vi "XOR Encryption - Stream Cipher.vi"() -> ()   [LabVIEW 2016]
uses:
  <extravilib>/ChannelInstances/Stream-str/Read With Abort.vi
  <extravilib>/ChannelInstances/Stream-str/Write With Abort.vi
  <extravilib>/ChannelInstances/Stream-str/EndpointRead.vi
  <extravilib>/ChannelInstances/Stream-str/Endpoint.vi
  <extravilib>/ChannelInstances/Stream-str/Instantiate.vi
  <extravilib>/ChannelInstances/Stream-str/)Channel.vi
  <resource>/ChannelSupport/_ChannelSupport/WaitIfNeeded.vi
  <extravilib>/ChannelInstances/Stream-str.lvlib
  <vilib>/Analysis/NI_AALBase.lvlib
panel:
  out "min value":u8
  out "max value":u8
  out "Key Distribution":dynamicdata(graph)=[{"t0"=timestamp(0.5 s since 1904-01-01), "dt"=1.0, "Y"=[5.0, 0.0, 5.0, 0.0, 2.0, 0.0, 2.0, 0.0, 3.0, 0.0, 4.0, 0.0, 3.0, 0.0, 1.0, 0.0, 2.0, 0.0, 4.0, 0.0, 6.0, 0.0, 2.0, 0.0, 1.0, 0.0, 1.0, 0.0, 4.0, 0.0, 5.0, 0.0, 5.0, 0.0, 5.0, 0.0, 4.0, 0.0, 1.0, 0.0, 6.0, 0.0, 4.0, 0.0, 5.0, 0.0, 3.0, 0.0, 6.0, 0.0, 2.0, 0.0, 2.0, 0.0, 0.0, 0.0, 3.0, 0.0, 4.0, 0.0, 2.0, 0.0, 4.0, 0.0, 4.0, 0.0, 5.0, 0.0, 2.0, 0.0, 3.0, 0.0, 3.0, 0.0, 0.0, 0.0, 3.0, 0.0, 5.0, 0.0, 1.0, 0.0, 0.0, 0.0, 1.0, 0.0, 6.0, 0.0, 4.0, 0.0, 9.0, 0.0, 7.0, 0.0, 6.0, 0.0, 6.0, 0.0, 5.0, 0.0, 6.0, 0.0, 1.0, 0.0, 8.0, 0.0, 4.0, 0.0, 5.0, 0.0, 3.0, 0.0, 6.0, 0.0, 7.0, 0.0, 7.0, 0.0, 4.0, 0.0, 4.0, 0.0, 0.0, 0.0, 5.0, 0.0, 3.0, 0.0, 1.0, 0.0, 5.0, 0.0, 4.0, 0.0, 2.0, 0.0, 3.0, 0.0, 5.0, 0.0, 5.0, 0.0, 3.0, 0.0, 5.0, 0.0, 1.0, 0.0, 3.0, 0.0, 2.0, 0.0, 3.0, 0.0, 6.0, 0.0, 2.0, 0.0, 4.0, 0.0, 4.0, 0.0, 3.0, 0.0, 1.0, 0.0, 4.0, 0.0, 3.0, 0.0, 3.0, 0.0, 5.0, 0.0, 2.0, 0.0, 1.0, 0.0, 3.0, 0.0, 4.0, 0.0, 3.0, 0.0, 2.0, 0.0, 1.0, 0.0, 4.0, 0.0, 3.0, 0.0, 6.0, 0.0, 2.0, 0.0, 8.0, 0.0, 1.0, 0.0, 4.0, 0.0, 2.0, 0.0, 2.0, 0.0, 2.0, 0.0, 6.0, 0.0, 3.0, 0.0, 2.0, 0.0, 3.0, 0.0, 5.0, 0.0, 2.0, 0.0, 3.0, 0.0, 5.0, 0.0, 3.0, 0.0, 5.0, 0.0, 2.0, 0.0, 1.0, 0.0, 3.0, 0.0, 3.0, 0.0, 3.0, 0.0, 0.0, 0.0, 4.0, 0.0, 4.0, 0.0, 4.0, 0.0, 6.0, 0.0, 3.0, 0.0, 4.0, 0.0, 4.0, 0.0, 1.0, 0.0], "attributes"=variant("NI_ChannelName"=variant(string " (Histogram)"), "NI_ExpIsRelativeTime"=variant(bool TRUE), "NI_ExpStartTimeStamp"=variant(timestamp timestamp(3588586549.4751897 s since 1904-01-01)), "NI_ExpTimeStamp"=variant(timestamp timestamp(3588586549.4751897 s since 1904-01-01)), "NI_ExpXDimension"=variant(string "BIN"), "NI_OriginalChannelName"=variant(string ""))}] caption="Histogram"
  out "Cypher Text":string
  out "Data Out":string
  in  "Plaintext":string
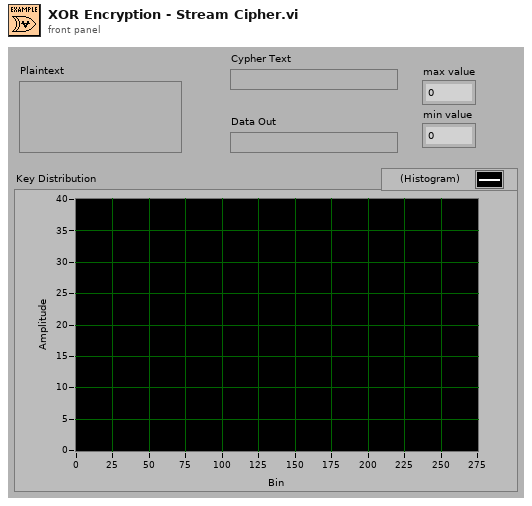
[diagram p1: front panel]
types:
  T1 = typedef "Stream-str.lvlib/)Channel.ctl" = refnum<queue>
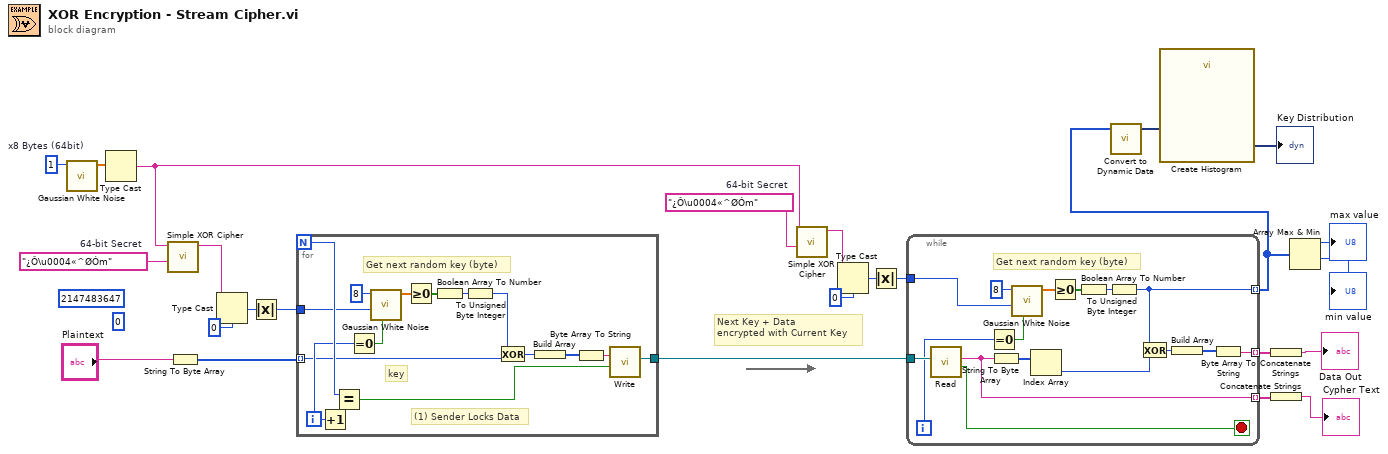
[diagram p0: block diagram]
diagram:
  (unwired) 0 ("seed")
  (unwired) 2147483647 ("seed")
  w14 = "¿Ô\u0004«^ØÓm"  # 64-bit Secret
  w15 = "¿Ô\u0004«^ØÓm"  # 64-bit Secret
  w18 = 1  # x8 Bytes (64bit)
  # "Next Key + Data\nencrypted with Current Key"
  n1 = call <vilib>:"Gaussian White Noise.vi"("samples"=w18) -> ("Gaussian noise pattern"=w17:dbl[])  [unwired: 9 in, 1 out]
  n2 = Type Cast(x=w17) -> (*(type *) &x=w16:string)  [unwired: 1 in]
  n3 = call "Simple XOR Cipher.vi"("key (\"\": random)"=w15, "data in"=w16) -> ("data out"=w13:string)  [unwired: 8 in, 1 out]
  n4 = String To Byte Array(string="Plaintext") -> (unsigned byte array=w22:u8[])
  n5 = Type Cast(type=0 ("seed"), x=w13) -> (*(type *) &x=w11:i32)
  n6 = Absolute Value(x=w11) -> (abs(x)=w7:i32)
  n7 = for {
    N -> [w40]
    tunnel: w22 -> [w34] mode=indexing
    tunnel: [w41] -> w24
    tunnel: w7 -> [w30]
    i -> [w36]
    # "Get next random key (byte)"
    # "key"
    # "(1) Sender Locks Data"
    n8 = Increment(x=w36) -> (x+1=w39:i32)
    n9 = Equal?(x=w40, y=w39) -> (x = y?=w38:bool)
    n10 = Equal To 0?(x=w36) -> (x = 0?=w35:bool)
    n11 = call <vilib>:"Gaussian White Noise.vi"("initialize?"=w35, "seed"=w30, "samples"=8) -> ("Gaussian noise pattern"=w27:dbl[])  [unwired: 7 in, 1 out]
    n12 = Greater Or Equal To 0?(x=w27) -> (x >= 0?=w29:bool[])
    n13 = Boolean Array To Number(Boolean array=w29) -> (number=w28:u32)
    n14 = To Unsigned Byte Integer(number=w28) -> (unsigned 8bit integer=w26:u8)
    n15 = Exclusive Or(1:w34, 2:w26) -> (0:w33:u8)
    n16 = Build Array(w33) -> (w31:u8[])
    n17 = Byte Array To String(unsigned byte array=w31) -> (string=w32:string)
    n18 = call <extravilib>:"Write.vi"("last element? (F)"=w38, "element"=w32) -> ("channel"=w41:T1)  [unwired: 7 in, 2 out]
  }
  n19 = call "Simple XOR Cipher.vi"("key (\"\": random)"=w14, "data in"=w16) -> ("data out"=w9:string)  [unwired: 8 in, 1 out]
  n20 = Type Cast(type=0 ("seed"), x=w9) -> (*(type *) &x=w8:i32)
  n21 = Absolute Value(x=w8) -> (abs(x)=w6:i32)
  n22 = while {
    tunnel: [w49] -> w25 mode=indexing
    tunnel: w24 -> [w57]
    tunnel: [w47] -> w20 mode=indexing
    tunnel: w6 -> [w46]
    tunnel: [w42] -> w3 mode=indexing
    i -> [w48]
    stop <- w56 stop-if-true
    # "Get next random key (byte)"
    n23 = call <extravilib>:"Read.vi"("channel"=w57) -> ("last element?"=w56:bool, "element"=w47:string)  [unwired: 6 in, 3 out]
    n24 = Equal To 0?(x=w48) -> (x = 0?=w54:bool)
    n25 = String To Byte Array(string=w47) -> (unsigned byte array=w51:u8[])
    n26 = call <vilib>:"Gaussian White Noise.vi"("initialize?"=w54, "seed"=w46, "samples"=8) -> ("Gaussian noise pattern"=w45:dbl[])  [unwired: 7 in, 1 out]
    n27 = Index Array(array=w51) -> (element=w50:u8)  [unwired: 1 in]
    n28 = Greater Or Equal To 0?(x=w45) -> (x >= 0?=w44:bool[])
    n29 = Boolean Array To Number(Boolean array=w44) -> (number=w43:u32)
    n30 = To Unsigned Byte Integer(number=w43) -> (unsigned 8bit integer=w42:u8)
    n31 = Exclusive Or(1:w50, 2:w42) -> (0:w53:u8)
    n32 = Build Array(w53) -> (w52:u8[])
    n33 = Byte Array To String(unsigned byte array=w52) -> (string=w49:string)
  }
  n34 = call "Convert to Dynamic Data"("Array"=w3) -> ("Dynamic Data Type"=w5:dynamicdata)  [unwired: 3 in]
  n35 = call "Create Histogram"("Signal"=w5) -> ("Histogram"=→"Key Distribution":dynamicdata)  [unwired: 9 in, 1 out]
  n36 = Concatenate Strings(w25) -> (→"Data Out":string)
  n37 = Concatenate Strings(w20) -> (→"Cypher Text":string)
  n38 = Array Max & Min(array=w3) -> (max value=→"max value":u8, min value=→"min value":u8)  [unwired: 2 out]
